vi "Simple cDAQ thermocouple with data logging example.vi"() -> ()   [LabVIEW 2015]
uses:
  <vilib>/express/express shared/transition.llb/Dynamic To Waveform Array.vi
  <vilib>/express/express signal manip/GetorSetDDTAttributes/Set DDT Attributes/SetT0.vi
  <vilib>/express/express shared/transition.llb/Waveform Array To Dynamic.vi
  <vilib>/express/express signal manip/GetorSetDDTAttributes/Set DDT Attributes/Set DDT Properties.xnode
panel:
  out "Stop loops":bool
  in  "stop":bool
  out "Temperature":dbl(graph)
  out "Loop counter":i32
  out "Temperature":dbl
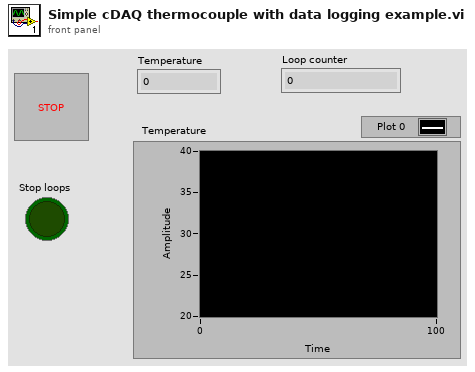
[diagram p1: front panel]
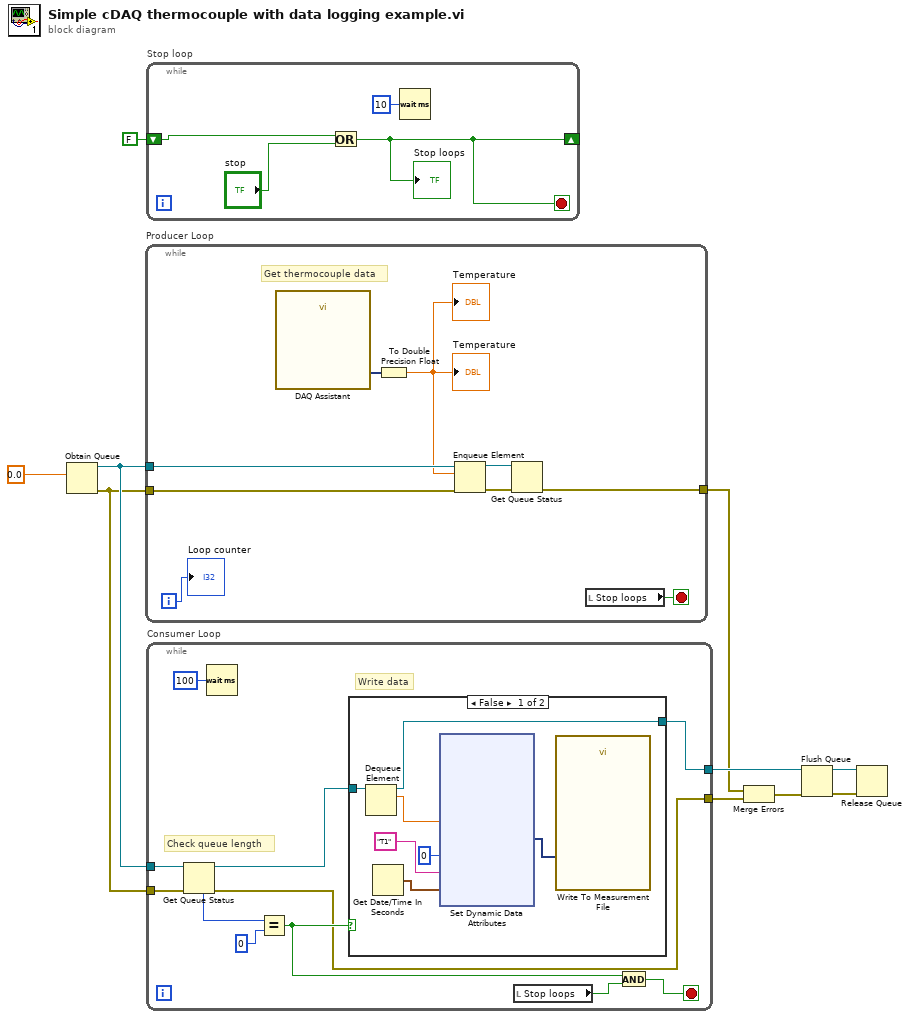
[diagram p0: block diagram]
diagram:
  n1 = Obtain Queue(element data type=0.0) -> (queue out=w8:refnum<queue>, error out=w4:errorcluster)  [unwired: 4 in, 1 out]
  n2 = while "Producer Loop" {
    tunnel: w8 -> [w17]
    tunnel: w4 -> [w13]
    tunnel: [w11] -> w5
    i -> [w19]
    stop <- w14 stop-if-true
    # "Get thermocouple data"
    n3 = call "DAQ Assistant"() -> ("data"=w18:dynamicdata)  [unwired: 16 in, 3 out]
    n4 = To Double Precision Float(number=w18) -> (double precision float=w16:dbl)
    "Temperature" <- w16
    "Temperature" <- w16
    n5 = Enqueue Element(queue=w17, element=w16, error in (no error)=w13) -> (queue out=w15:refnum<queue>, error out=w12:errorcluster)  [unwired: 1 in, 1 out]
    n6 = Get Queue Status(queue=w15, error in (no error)=w12) -> (error out=w11:errorcluster)  [unwired: 1 in, 7 out]
    n7 = local read "Stop loops"() -> (w14:bool)
    "Loop counter" <- w19
  }
  n8 = while "Stop loop" {
    shift-right: [w21] -> _
    shift-left: FALSE -> [w22]
    stop <- w21 stop-if-true
    n9 = Or(x=w22, y="stop") -> (x .or. y?=w21:bool)
    "Stop loops" <- w21
    n10 = Wait (ms)(milliseconds to wait=u32 10) -> ()  [unwired: 1 out]
  }
  n11 = while "Consumer Loop" {
    tunnel: w8 -> [w30]
    tunnel: [w26] -> w6
    tunnel: w4 -> [w25]
    tunnel: [w24] -> w3
    stop <- w31 stop-if-true
    # "Write data"
    # "Check queue length"
    n12 = Get Queue Status(queue=w30, error in (no error)=w25) -> (queue out=w27:refnum<queue>, error out=w24:errorcluster, # elements in queue=w34:i32)  [unwired: 1 in, 5 out]
    n13 = Wait (ms)(milliseconds to wait=u32 100) -> ()  [unwired: 1 out]
    n14 = Equal?(x=w34, y=0) -> (x = y?=w29:bool)
    n15 = case shown="False" w29 {
      tunnel: w27 -> [w36 w59]
      tunnel: [w35 w59] -> w26
      frame False {
        n16 = Dequeue Element(queue=w36) -> (queue out=w35:refnum<queue>, element=w37:dbl)  [unwired: 2 in, 2 out]
        n17 = Get Date/Time In Seconds() -> (seconds since 1Jan1904=w40:timestamp)
        n18 = xnode "Set Dynamic Data Attributes"("Signals In"=w37, "Signal Index"=0, "Signal Name"="T1", "Timestamp"=w40) -> ("Signals Out"=w39:dynamicdata)  [unwired: 1 in, 1 out]
        n19 = call "Write To Measurement File"("Signals"=w39) -> ()  [unwired: 16 in, 3 out]
      }
      frame True {
      }
    }
    n20 = local read "Stop loops"() -> (w32:bool)
    n21 = And(x=w29, y=w32) -> (x .and. y?=w31:bool)
  }
  n22 = Merge Errors(w5, w3) -> (w2:errorcluster)
  n23 = Flush Queue(queue=w6, error in (no error)=w2) -> (queue out=w7:refnum<queue>, error out=w1:errorcluster)  [unwired: 1 out]
  n24 = Release Queue(queue=w7, error in (no error)=w1) -> ()  [unwired: 1 in, 3 out]
